vi "读取excel中的数据.vi"(8 "错误输入（无错误）":errorcluster, 10 "表单索引":variant, 11 "excel路径":path) -> (0 "错误输出":errorcluster, 3 "excel数值":string[][](array[string]))   [LabVIEW 2013, in "excel处理.lvlib"]
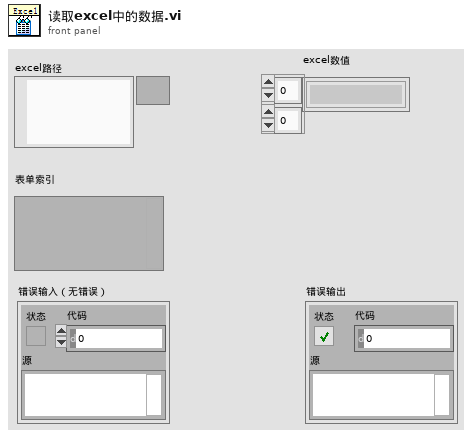
[diagram p1: front panel]
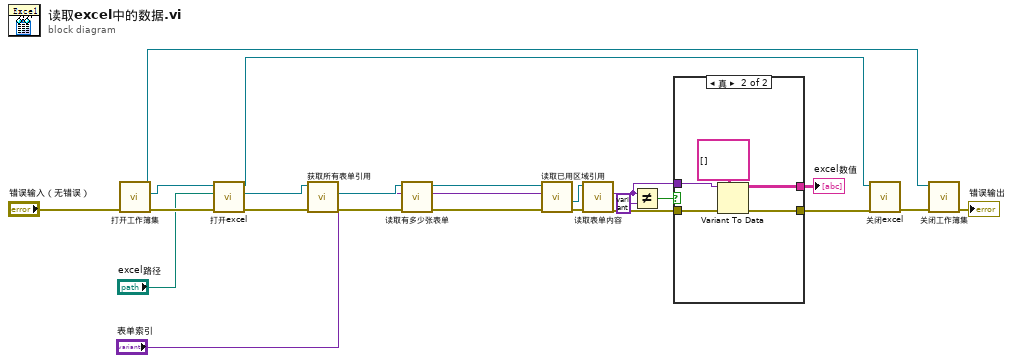
[diagram p0: block diagram]
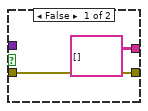
[diagram p2: hidden frame]
diagram:
  n1 = call "打开工作簿集.vi"("错误输入（无错误）"="错误输入（无错误）") -> ("错误输出"=w23:errorcluster, "工作簿集"=w18:refnum<k7>, "excel.application输出"=w13:refnum<k7>)  [unwired: 8 in]
  n2 = call "打开excel.vi"("错误输入（无错误）"=w23, "excel路径"="excel路径", "工作簿引用"=w18) -> ("错误输出"=w22:errorcluster, "excel引用"=w17:refnum<k7>, "工作簿输出"=w14:refnum<k7>)  [unwired: 6 in]
  n3 = call "获取所有表单引用.vi"("错误输入（无错误）"=w22, "excel引用"=w17) -> ("错误输出"=w21:errorcluster, "Worksheets"=w16:refnum<k7>)  [unwired: 7 in, 1 out]
  n4 = call "读取有多少张表单.vi"("错误输入（无错误）"=w21, "所有表单引用"=w16) -> ("错误输出"=w20:errorcluster, "所有表单引用输出"=w15:refnum<k7>)  [unwired: 7 in, 1 out]
  n5 = call "读取已用区域引用.vi"("错误输入（无错误）"=w20, "表单索引"="表单索引", "所有表单引用"=w15) -> ("错误输出"=w9:errorcluster, "选中引用输出"=w8:refnum<k7>)  [unwired: 5 in, 2 out]
  n6 = call "读取表单内容.vi"("错误输入（无错误）"=w9, "选中区域引用输入"=w8) -> ("错误输出"=w4:errorcluster, "数值"=w2:variant)  [unwired: 7 in, 1 out]
  n7 = Not Equal?(x=w2, y=variant) -> (x != y?=w5:bool)
  n8 = case shown="真" w5 {
    tunnel: w4 -> [w25 w29]
    tunnel: [w25 w28] -> w3
    tunnel: [string[][] [] w27] -> w1
    tunnel: w2 -> [_ w26]
    frame False {
    }
    frame True {
      n9 = Variant To Data(error in=w29, type=string[][] [], Variant=w26) -> (data=w27:string[][], error out=w28:errorcluster)
    }
  }
  "excel数值" <- w1
  n10 = call "关闭excel.vi"("错误输入（无错误）"=w3, "引用"=w14) -> ("错误输出"=w19:errorcluster)  [unwired: 8 in, 1 out]
  n11 = call "关闭工作簿集.vi"("错误输入（无错误）"=w19, "工作薄引用"=w13) -> ("错误输出"=→"错误输出":errorcluster)  [unwired: 8 in, 1 out]
